vi "VISA update settings.vi"(8 "error in (no error)":errorcluster, 11 "AOTF in":refnum<class "AOTF.lvclass">) -> (0 "error out":errorcluster, 3 "AOTF out":refnum<class "AOTF.lvclass">)   [LabVIEW 2012, in "AOTF.lvclass"]
uses:
  AOTF.lvclass
  AOTF.lvclass/AOTF.ctl
panel:
  out "concatenated string":string
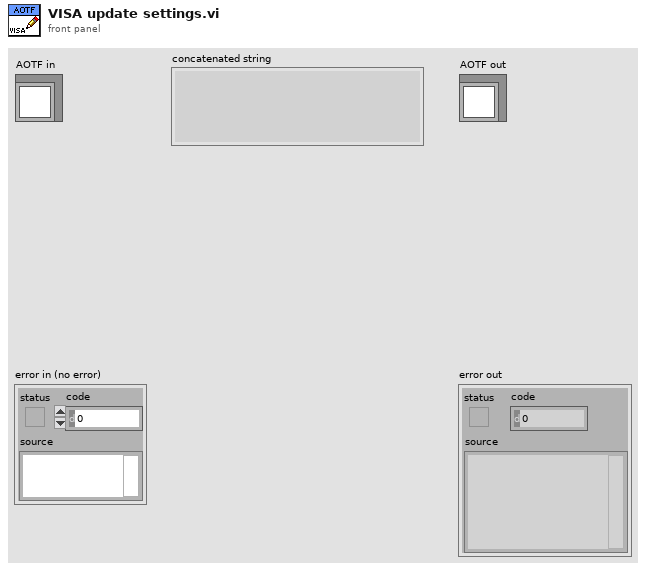
[diagram p1: front panel]
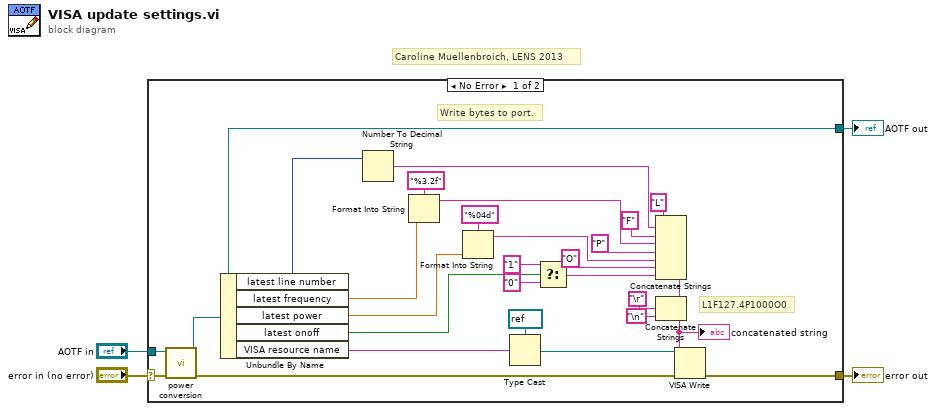
[diagram p0: block diagram]
diagram:
  # "Caroline Muellenbroich, LENS 2013"
  n1 = case shown="No Error" "error in (no error)" {
    selector: "error in (no error)" -> [w8 w34]
    tunnel: [w21 w34] -> w3
    tunnel: [w5 w33] -> w1
    tunnel: "AOTF in" -> [w6 w33]
    frame No Error {
      # "L1F127.4P1000O0"
      # "Write bytes to port."
      n2 = call-dynamic "power conversion.vi"("error in (no error)"=w8, "AOTF in"=w6) -> ("error out"=w7:errorcluster, "AOTF out"=w5:refnum<class "AOTF.lvclass">)  [unwired: 8 in]
      n3 = Unbundle By Name(w5) -> ("latest line number"=w20:i32, "latest frequency"=w18:dbl, "latest power"=w15:dbl, "latest onoff"=w9:bool, "VISA resource name"=w24:string)
      n4 = Number To Decimal String(number=w20) -> (decimal integer string=w22:string)  [unwired: 1 in]
      n5 = Format Into String(format string="%3.2f", w18) -> (resulting string=w16:string)  [unwired: 2 in, 1 out]
      n6 = Format Into String(format string="%04d", w15) -> (resulting string=w14:string)  [unwired: 2 in, 1 out]
      n7 = Type Cast(type=refnum<visa-resource-name> refnum ("VISA resource name"), x=w24) -> (*(type *) &x=w19:refnum<visa-resource-name>)
      n8 = Select(t="1" ("string"), s=w9, f="0" ("string")) -> (s? t:f=w12:string)
      n9 = Concatenate Strings("L", w22, "F" ("string"), w16, "P" ("string"), w14, "O" ("string"), w12) -> (w32:string)
      n10 = Concatenate Strings(w32, "\r", "\n") -> (w26:string)
      "concatenated string" <- w26
      n11 = VISA Write(VISA resource name=w19, write buffer=w26, error in (no error)=w7) -> (error out=w21:errorcluster)  [unwired: 2 out]
    }
    frame Error {
    }
  }
  "error out" <- w3
  "AOTF out" <- w1
